vi "HCC Panel Get Cycle Count.vi"(0 "Main Washer Display In":T9={"Status Color"=0, "Station Label Display"="", "Cycle Count Display"=0, "Board ID Display"="", "Serial Number Display"="", "Current Display"=0.0, "RPM Display"=0, "Saving Display"=FALSE, "Appliance Details"={"FileVersionInfo"={"FileVersion"="", "ProductName"="", "InternalName"="", "CompanyName"="", "LegalCopyright"="", "FileDescription"=""}, "Dishwasher Info"={"Open Cup Weight (gm):"=0.0, "Auto Cup Weight (gm):"=0.0, "Detergent-Dish:"="", "Inlet Temperature-Dish:"="", "Cycle Mode-Dish:"="", "Unit Control-Dish:"="", "Manufacturer-Dish:"=""}, "Washer Info"={"Hot Water Temperature (Fahrenheit):"="", "Cold Water Temperature (Fahrenheit):"="", "Capacity (cu.ft):"=0.0, "Initial Cloth Weight:"=0.0, "Cloth Lot:"=0, "Model Family:"="", "Program Name:"="", "Cycle Selection:"="", "Wash Temperature:"="", "Rinse Temperature:"="", "Load Size:"=""}, "File Name Output Array"=[], "Calibration Output Array"=[], "Appliance Common"={"Engineer:"="", "Model Number:"="", "Serial Number:"="", "Comments:"="", "Station ID:"="", "Technician:"="", "TR Number:"="", "Lab ID:"="", "Voltage:"="", "Water Pressure (PSI):"="", "Test Date:"="", "Computer Name:"="", "IP Address:"="", "Ambient RH:"="", "Frequency:"="", "Build:"="", "Filename:"="", "Test Type:"="", "Load Run #:"=0, "Ambient Temperature (F):"="", "File Path:"=path ""}, "Water Heater"={"Heating Mode:"=""}, "Dryer"={"Heat Setting:"="", "Washer Water Temperature (60 ± 5°F):"=60, "Water Hardness (PPM):"=17, "Dryness Setting:"="", "Dryer Type:"="", "Exhaust:"="", "Drying Cycle:"="", "Load Type:"="", "Nominal Load Weight"="", "Dryer Initial IMC Data"={"Measured IMC"=7.0, "Actual RMC"=7.0, "RMC (Desired)"=100.0, "Bone Dry Wt(lbs)"=7.0, "Tolerance(%)"=5.0}, "Empty Dryer Cold Weigth"=60.0}}, "Current Run Start Time Display"=0.0, "UI Button"=FALSE, "Current Path Display"=path "", "Unit Type Display"=enum."", "Total Time On Display"=0.0, "Headers"={"Summary Header"=["Date", "Time", "Total Cycle Time (Seconds)", "Cycle Number", "Maximum RPM", "# of Error Codes", "Maximum Current"], "Current Header"=["Date", "Time", "Time (Seconds)", "Current (Amps)"], "Debug Log Header"=["Date", "Time", "Debug Logs"], "Data Header"=["Date", "Time", "Time (Seconds)", "IGBT Temperature", "Speed", "Load Size", "Temperature", "Water Pressure", "Detergent", "Fabric Softener", "Direction", "Detergent Valve", "Fabric Softener Valve", "Recirculating Pump", "Drain Valve", "Hot Water Valve", "Cold Water Valve", "Lid Status", "Lid Lock Status", "Machine Status", "Serial Number", "Cycle Count", "Station Label", "Board ID", "Error", "End of Cycle"]}} {"Appliance Details"."Dryer"."Dryer Initial IMC Data"."Tolerance(%)" format="%0#_6g"; "Appliance Details"."Dryer"."Dryer Initial IMC Data"."Bone Dry Wt(lbs)" format="%03_6g"; "Appliance Details"."Dryer"."Dryer Initial IMC Data"."RMC (Desired)" format="%0#_6g"; "Appliance Details"."Dryer"."Dryer Initial IMC Data"."Actual RMC" format="%03_6g"; "Appliance Details"."Dryer"."Dryer Initial IMC Data"."Measured IMC" format="%0#_6g"; "Current Display" format="%.2f"; "Cycle Count Display" format="%04d"}, 2 "GEA Information In":T1 {"Water Heater GEA2 Data"."Hyperterminal Data"."CRC" format="%x"; "Water Heater GEA2 Data"."Hyperterminal Data"."Length" format="%x"; "Water Heater GEA2 Data"."Hyperterminal Data"."Command" format="%x"; "Water Heater GEA2 Data"."Hyperterminal Data"."Destination" format="%x"; "Water Heater GEA2 Data"."Hyperterminal Data"."Source" format="%x"; "Destination Address" format="%x"; "Source Address" format="%x"; "Command" format="%.0x"; "Data to send" format="%x"; "ReceivedData" format="%x"}, 5 "error in (no error)":errorcluster) -> (14 "Main Washer Display Out":T9={"Status Color"=0, "Station Label Display"="", "Cycle Count Display"=0, "Board ID Display"="", "Serial Number Display"="", "Current Display"=0.0, "RPM Display"=0, "Saving Display"=FALSE, "Appliance Details"={"FileVersionInfo"={"FileVersion"="", "ProductName"="", "InternalName"="", "CompanyName"="", "LegalCopyright"="", "FileDescription"=""}, "Dishwasher Info"={"Open Cup Weight (gm):"=0.0, "Auto Cup Weight (gm):"=0.0, "Detergent-Dish:"="", "Inlet Temperature-Dish:"="", "Cycle Mode-Dish:"="", "Unit Control-Dish:"="", "Manufacturer-Dish:"=""}, "Washer Info"={"Hot Water Temperature (Fahrenheit):"="", "Cold Water Temperature (Fahrenheit):"="", "Capacity (cu.ft):"=0.0, "Initial Cloth Weight:"=0.0, "Cloth Lot:"=0, "Model Family:"="", "Program Name:"="", "Cycle Selection:"="", "Wash Temperature:"="", "Rinse Temperature:"="", "Load Size:"=""}, "File Name Output Array"=[], "Calibration Output Array"=[], "Appliance Common"={"Engineer:"="", "Model Number:"="", "Serial Number:"="", "Comments:"="", "Station ID:"="", "Technician:"="", "TR Number:"="", "Lab ID:"="", "Voltage:"="", "Water Pressure (PSI):"="", "Test Date:"="", "Computer Name:"="", "IP Address:"="", "Ambient RH:"="", "Frequency:"="", "Build:"="", "Filename:"="", "Test Type:"="", "Load Run #:"=0, "Ambient Temperature (F):"="", "File Path:"=path ""}, "Water Heater"={"Heating Mode:"=""}, "Dryer"={"Heat Setting:"="", "Washer Water Temperature (60 ± 5°F):"=60, "Water Hardness (PPM):"=17, "Dryness Setting:"="", "Dryer Type:"="", "Exhaust:"="", "Drying Cycle:"="", "Load Type:"="", "Nominal Load Weight"="", "Dryer Initial IMC Data"={"Measured IMC"=7.0, "Actual RMC"=7.0, "RMC (Desired)"=100.0, "Bone Dry Wt(lbs)"=7.0, "Tolerance(%)"=5.0}, "Empty Dryer Cold Weigth"=60.0}}, "Current Run Start Time Display"=0.0, "UI Button"=FALSE, "Current Path Display"=path "", "Unit Type Display"=enum."", "Total Time On Display"=0.0, "Headers"={"Summary Header"=["Date", "Time", "Total Cycle Time (Seconds)", "Cycle Number", "Maximum RPM", "# of Error Codes", "Maximum Current"], "Current Header"=["Date", "Time", "Time (Seconds)", "Current (Amps)"], "Debug Log Header"=["Date", "Time", "Debug Logs"], "Data Header"=["Date", "Time", "Time (Seconds)", "IGBT Temperature", "Speed", "Load Size", "Temperature", "Water Pressure", "Detergent", "Fabric Softener", "Direction", "Detergent Valve", "Fabric Softener Valve", "Recirculating Pump", "Drain Valve", "Hot Water Valve", "Cold Water Valve", "Lid Status", "Lid Lock Status", "Machine Status", "Serial Number", "Cycle Count", "Station Label", "Board ID", "Error", "End of Cycle"]}} {"Appliance Details"."Dryer"."Dryer Initial IMC Data"."Tolerance(%)" format="%0#_6g"; "Appliance Details"."Dryer"."Dryer Initial IMC Data"."Bone Dry Wt(lbs)" format="%03_6g"; "Appliance Details"."Dryer"."Dryer Initial IMC Data"."RMC (Desired)" format="%0#_6g"; "Appliance Details"."Dryer"."Dryer Initial IMC Data"."Actual RMC" format="%03_6g"; "Appliance Details"."Dryer"."Dryer Initial IMC Data"."Measured IMC" format="%0#_6g"; "Current Display" format="%.2f"; "Cycle Count Display" format="%04d"}, 16 "GEA Information Out":T1 {"Water Heater GEA2 Data"."Hyperterminal Data"."CRC" format="%x"; "Water Heater GEA2 Data"."Hyperterminal Data"."Length" format="%x"; "Water Heater GEA2 Data"."Hyperterminal Data"."Command" format="%x"; "Water Heater GEA2 Data"."Hyperterminal Data"."Destination" format="%x"; "Water Heater GEA2 Data"."Hyperterminal Data"."Source" format="%x"; "Destination Address" format="%x"; "Source Address" format="%x"; "Command" format="%.0x"; "Data to send" format="%x"; "ReceivedData" format="%x"}, 17 "GEA Ref Out":refnum<k24>, 18 "Event Registration Out":refnum<event-registration>, 19 "error out":errorcluster)   [LabVIEW 2014]
uses:
  Utility/Save File/Public/Type Definitions/Save File Washer.ctl
  Utility/Save File/File Setup (Public)/Type Definition/Save File DISH Dishwasher Details.ctl
  <vilib>/Platform/fileVersionInfo.llb/FileVersionInformation.ctl
  Utility/Custom Pallet Controls/Custom Pallet String.ctl
  Utility/Save File/Public/Type Definitions/Save File Unit Type.ctl
  Utility/Save File/Public/Type Definitions/Save File Headers.ctl
  Type Definitions/ViperHawk/ViperHawk Data.ctl
  Type Definitions/ViperHawk/ViperHawk Diagnostic Data.ctl
  Utility/Save File/Public/Type Definitions/Save File Software Version.ctl
  Type Definitions/ViperHawk/ViperHawk Search Control.ctl
  C:/Technology Lab/NI-2010/Trunk/Utility/LabVIEW GEA2 Toolkit v1.0.0.0/Appliance.NET/GeaCommunication.dll
  Utility/LabVIEW GEA2 Toolkit v1.0.0.0/Appliance.NET/GeaCommunication.dll
  Utility/LabVIEW GEA2 Toolkit v1.0.0.0/type defs/Data Out.ctl
  Utility/GEA2 Commands/HEWH/Type Definitions/GEA2 Commands WaterHeater GEA2 Data.ctl
  Utility/GEA2 Commands/HEWH/Type Definitions/GEA2 Commands Button Status.ctl
  Utility/GEA2 Commands/HEWH/Type Definitions/GEA2 Commands Status Query.ctl
  Utility/GEA2 Commands/HEWH/Type Definitions/GEA2 Commands Service Error Codes.ctl
  Utility/LabVIEW GEA2 Toolkit v1.0.0.0/type defs/ERD Read Data In.ctl
  Utility/LabVIEW GEA2 Toolkit v1.0.0.0/type defs/Data Type.ctl
  Utility/LabVIEW GEA2 Toolkit v1.0.0.0/type defs/Source_Destination.ctl
  Utility/LabVIEW GEA2 Toolkit v1.0.0.0/type defs/Data In.ctl
  Utility/LabVIEW GEA2 Toolkit v1.0.0.0/library/GEA2_Toolkit.lvlib
  Utility/Save File/Save File.lvlib
  Utility/Save File/File Setup.lvlib
panel:
  out "Total Cycle Count":u16
  in  "Complete":bool
  in  "String":string="Finding Machine Cycle Count"
  in  "Tab Control":enum32{"Page 1"}(tab)
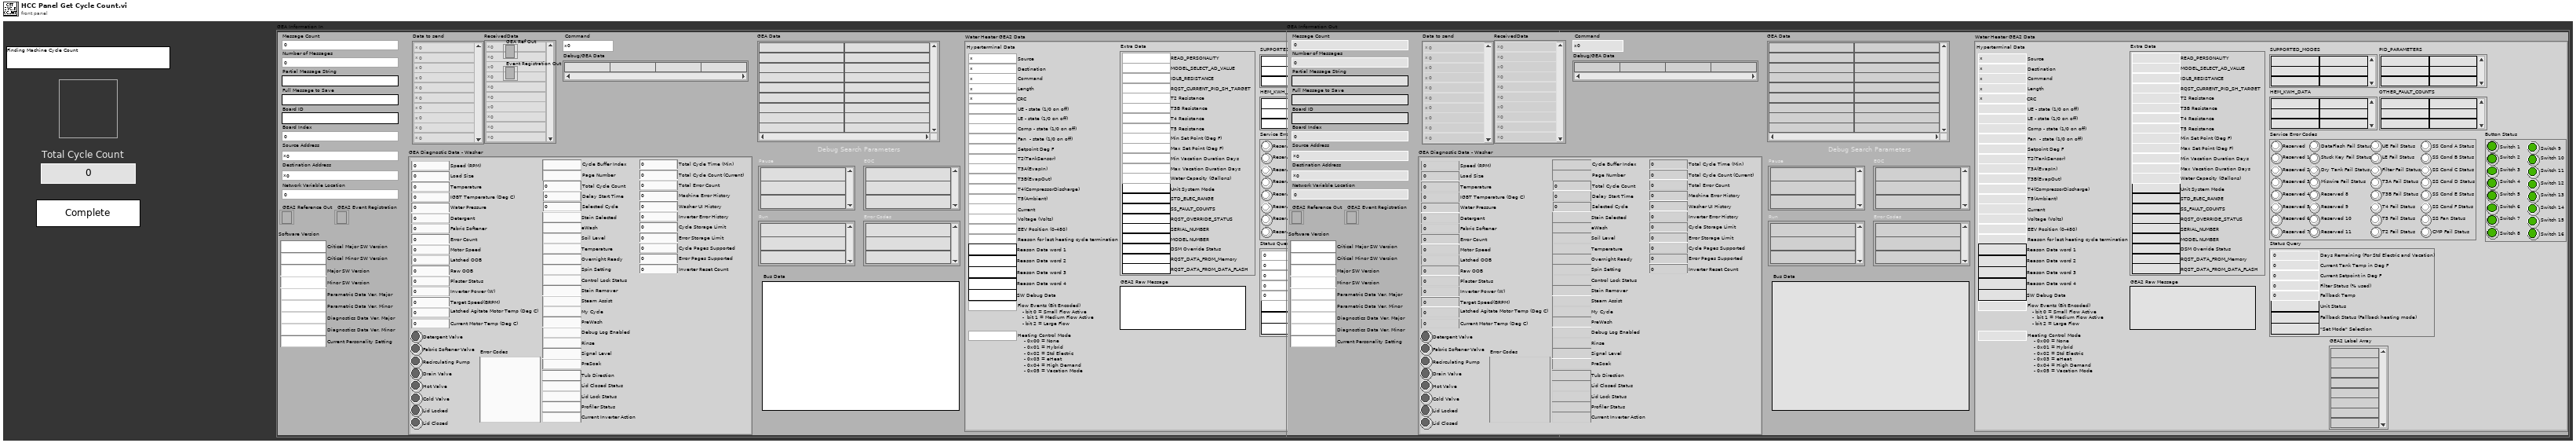
[diagram p1: front panel]
types:
  T1 = typedef "ViperHawk Data.ctl" = cluster{"GEA Diagnostic Data - Washer":T2, "Software Version":T3, "Debug Search Parameters":T4, "Message Count":i32, "Number of Messages":i32, "Partial Message String":string, "Full Message to Save":string, "Board ID":string, "Board Index":i32, "Source Address":u8, "Destination Address":u8, "Data to send":u8[], "ReceivedData":u8[], "Debug/GEA Data":string[], "Command":u8, "GEA2 Reference Out":refnum<k24>, "GEA2 Event Registration":refnum<event-registration>, "Bus Data":string, "GEA Data":string[][], "Network Variable Location":i32, "Water Heater GEA2 Data":T5}
  T2 = typedef "ViperHawk Diagnostic Data.ctl" = cluster{"Speed (RPM)":u32, "Load Size":u32, "Temperature":u32, "Water Pressure":u32, "Detergent":u32, "Fabric Softener":u32, "Tub Direction":string, "Detergent Valve":bool, "Fabric Softener Valve":bool, "Recirculating Pump":bool, "Drain Valve":bool, "Hot Valve":bool, "Cold Valve":bool, "Lid Closed Status":string, "Lid Lock Status":string, "Error Count":u32, "IGBT Temperature (Deg C)":u32, "Motor Speed":u32, "Latched OOB":u32, "Raw OOB":u32, "Plaster Status":u32, "Inverter Power (W)":u32, "Target Speed(BRPM)":u32, "Latched Agitate Motor Temp (Deg C)":u32, "Current Motor Temp (Deg C)":u32, "Profiler Status":string, "Current Inverter Action":string, "Error Codes":string, "Lid Locked":bool, "Lid Closed":bool, "9E Diagnostic Data":cluster{"Total Cycle Time (Min)":u32, "Total Cycle Count (Current)":u16, "Total Error Count":u16, "Machine Error History":u32, "Washer UI History":u32, "Inverter Error History":u32, "Cycle Storage Limit":u8, "Error Storage Limit":u8, "Cycle Pages Supported":u8, "Error Pages Supported":u8, "Inverter Reset Count":u16}, "9F Diagnostic Data":cluster{"Cycle Buffer Index":string, "Page Number":string, "Total Cycle Count":u32, "Delay Start Time":u32, "Stain Selected":string, "Selected Cycle":u32, "eWash":string, "Soil Level":string, "Temperature":string, "Overnight Ready":string, "Spin Setting":string, "Control Lock Status":string, "Stain Remover":string, "Steam Assist":string, "My Cycle":string, "PreWash":string, "Debug Log Enabled":string, "Rinse":string, "Signal Level":string, "PreSoak":string}}
  T3 = typedef "Save File.lvlib/Save File Software Version.ctl" = cluster{"Critical Major SW Version":string, "Critical Minor SW Version":string, "Major SW Version":string, "Minor SW Version":string, "Parametric Data Ver. Major":string, "Parametric Data Ver. Minor":string, "Diagnostics Data Ver. Major":string, "Diagnostics Data Ver. Minor":string, "Current Personality Setting":string}
  T4 = typedef "ViperHawk Search Control.ctl" = cluster{"Pause":string[], "Run":string[], "EOC":string[], "Error Codes":string[]}
  T5 = typedef "GEA2 Commands WaterHeater GEA2 Data.ctl" = cluster{"GEA2 Label Array":string[], "PID_PARAMETERS":string[][], "SUPPORTED_MODES":string[][], "Button Status":T6, "Status Query":T7, "Service Error Codes":T8, "HEM_KWH_DATA":string[][], "OTHER_FAULT_COUNTS":string[][], "GEA2 Raw Message":string, "Hyperterminal Data":cluster{"Source":u8, "Destination":u8, "Command":u8, "Length":u8, "CRC":u16, "UE - state (1/0 on off)":u8, "LE - state (1/0 on off)":u8, "Comp - state (1/0 on off)":u8, "Fan  - state (1/0 on off)":u8, "Setpoint Deg F":i32, "T2(TankSensor)":dbl, "T3A(EvapIn)":dbl, "T3B(EvapOut)":dbl, "T4(CompressorDischarge)":dbl, "T5(Ambient)":dbl, "Current":dbl, "Voltage (Volts)":u16, "EEV Position (0-480)":u16, "Reason for last heating cycle termination":u16, "Reason Data word 1":string, "Reason Data word 2":string, "Reason Data word 3":string, "Reason Data word 4":string, "SW Debug Data":string, "Flow Events (Bit Encoded)":u16, "Heating Control Mode":u16}, "Extra Data":cluster{"Water Capacity (Gallons)":u32, "Max Vacation Duration Days":u32, "Min Vacation Duration Days":u32, "Max Set Point (Deg F)":u32, "Min Set Point (Deg F)":u32, "T5 Resistance":u32, "T4 Resistance":u32, "T3B Resistance":u32, "T2 Resistance":u32, "STD_ELEC_RANGE":string, "SS_FAULT_COUNTS":string, "SERIAL_NUMBER":string, "READ_PERSONALITY":u8, "RQST_OVERRIDE_STATUS":string, "MODEL_SELECT_AD_VALUE":u32, "MODEL NUMBER":string, "IDLB_RESISTANCE":u32, "DSM Override Status":string, "RQST_DATA_FROM_Memory":string, "RQST_DATA_FROM_DATA_FLASH":string, "RQST_CURRENT_PID_SH_TARGET":u16, "Unit System Mode":string}}
  T6 = typedef "GEA2 Commands Button Status.ctl" = cluster{"Switch 1":bool, "Switch 2":bool, "Switch 3":bool, "Switch 4":bool, "Switch 5":bool, "Switch 6":bool, "Switch 7":bool, "Switch 8":bool, "Switch 9":bool, "Switch 10":bool, "Switch 11":bool, "Switch 12":bool, "Switch 13":bool, "Switch 14":bool, "Switch 15":bool, "Switch 16":bool}
  T7 = typedef "GEA2 Commands Status Query.ctl" = cluster{"Days Remaining (For Std Electric and Vacation)":u8, "Unit Status":string, "Current Tank Temp in Deg F":u8, "Current Setpoint in Deg F":u8, "Filter Status (% used)":u8, "Fallback Status (Fallback heating mode)":string, "Fallback Temp":u8, "\"Set Mode\" Selection":string}
  T8 = typedef "GEA2 Commands Service Error Codes.ctl" = cluster{"Reserved":bool, "Reserved 1":bool, "Reserved 2":bool, "Reserved 3":bool, "Reserved 4":bool, "Reserved 5":bool, "Reserved 6":bool, "Reserved 7":bool, "DataFlash Fail Status":bool, "Stuck Key Fail Status":bool, "Dry Tank Fail Status":bool, "Miswire Fail Status":bool, "Reserved 8":bool, "Reserved 9":bool, "Reserved 10":bool, "Reserved 11":bool, "UE Fail Status":bool, "LE Fail Status":bool, "Filter Fail Status":bool, "T3A Fail Status":bool, "T3B Fail Status":bool, "T4 Fail Status":bool, "T5 Fail Status":bool, "T2 Fail Status":bool, "SS Cond A Status":bool, "SS Cond B Status":bool, "SS Cond C Status":bool, "SS Cond D Status":bool, "SS Cond E Status":bool, "SS Cond F Status":bool, "SS Fan Status":bool, "CMP Fail Status":bool}
  T9 = typedef "Save File.lvlib/Save File Washer.ctl" = cluster{"Status Color":u32, "Station Label Display":string, "Cycle Count Display":i32, "Board ID Display":string, "Serial Number Display":string, "Current Display":dbl, "RPM Display":u32, "Saving Display":bool, "Appliance Details":T10, "Current Run Start Time Display":dbl, "UI Button":bool, "Current Path Display":path, "Unit Type Display":T13, "Total Time On Display":dbl, "Headers":T14}
  T10 = typedef "File Setup.lvlib/Save File DISH Dishwasher Details.ctl" = cluster{"FileVersionInfo":T11, "Dishwasher Info":cluster{"Open Cup Weight (gm):":dbl, "Auto Cup Weight (gm):":dbl, "Detergent-Dish:":string, "Inlet Temperature-Dish:":string, "Cycle Mode-Dish:":string, "Unit Control-Dish:":string, "Manufacturer-Dish:":string}, "Washer Info":cluster{"Hot Water Temperature (Fahrenheit):":string, "Cold Water Temperature (Fahrenheit):":string, "Capacity (cu.ft):":dbl, "Initial Cloth Weight:":dbl, "Cloth Lot:":i32, "Model Family:":string, "Program Name:":string, "Cycle Selection:":string, "Wash Temperature:":string, "Rinse Temperature:":string, "Load Size:":string}, "File Name Output Array":string[][], "Calibration Output Array":string[][], "Appliance Common":cluster{"Engineer:":string, "Model Number:":string, "Serial Number:":string, "Comments:":string, "Station ID:":string, "Technician:":string, "TR Number:":string, "Lab ID:":string, "Voltage:":string, "Water Pressure (PSI):":string, "Test Date:":string, "Computer Name:":string, "IP Address:":string, "Ambient RH:":string, "Frequency:":string, "Build:":string, "Filename:":string, "Test Type:":string, "Load Run #:":i32, "Ambient Temperature (F):":string, "File Path:":path}, "Water Heater":cluster{"Heating Mode:":string}, "Dryer":cluster{"Heat Setting:":T12, "Washer Water Temperature (60 ± 5°F):":u16, "Water Hardness (PPM):":u16, "Dryness Setting:":T12, "Dryer Type:":string, "Exhaust:":string, "Drying Cycle:":string, "Load Type:":string, "Nominal Load Weight":string, "Dryer Initial IMC Data":cluster{"Measured IMC":dbl, "Actual RMC":dbl, "RMC (Desired)":dbl, "Bone Dry Wt(lbs)":dbl, "Tolerance(%)":dbl}, "Empty Dryer Cold Weigth":dbl}}
  T11 = typedef "FileVersionInformation.ctl" = cluster{"FileVersion":string, "ProductName":string, "InternalName":string, "CompanyName":string, "LegalCopyright":string, "FileDescription":string}
  T12 = typedef "Custom Pallet String.ctl" = string
  T13 = typedef "Save File.lvlib/Save File Unit Type.ctl" = enum32{"", "Viper", "Hawk", "2015", "HEWH", "Other"}
  T14 = typedef "Save File Headers.ctl" = cluster{"Summary Header":string[], "Current Header":string[], "Debug Log Header":string[], "Data Header":string[]}
  T15 = typedef "GEA2_Toolkit.lvlib/Data In.ctl" = cluster{"Source":u8, "Destination":u8, "Command":u8, "Message":string}
  T16 = typedef "GEA2_Toolkit.lvlib/Source_Destination.ctl" = cluster{"Source":u8, "Destination":u8}
  T17 = typedef "GEA2_Toolkit.lvlib/ERD Read Data In.ctl" = cluster{"ERD Number":u16, "Data Type":T18}
  T18 = typedef "GEA2_Toolkit.lvlib/Data Type.ctl" = enum16{"string", "boolean", "uint8_t", "uint16_t", "uint32_t", "uint64_t"}
  T19 = typedef "GEA2_Toolkit.lvlib/ERD Read Data Out.ctl" = cluster{"ERD Number":u16, "Data":string}
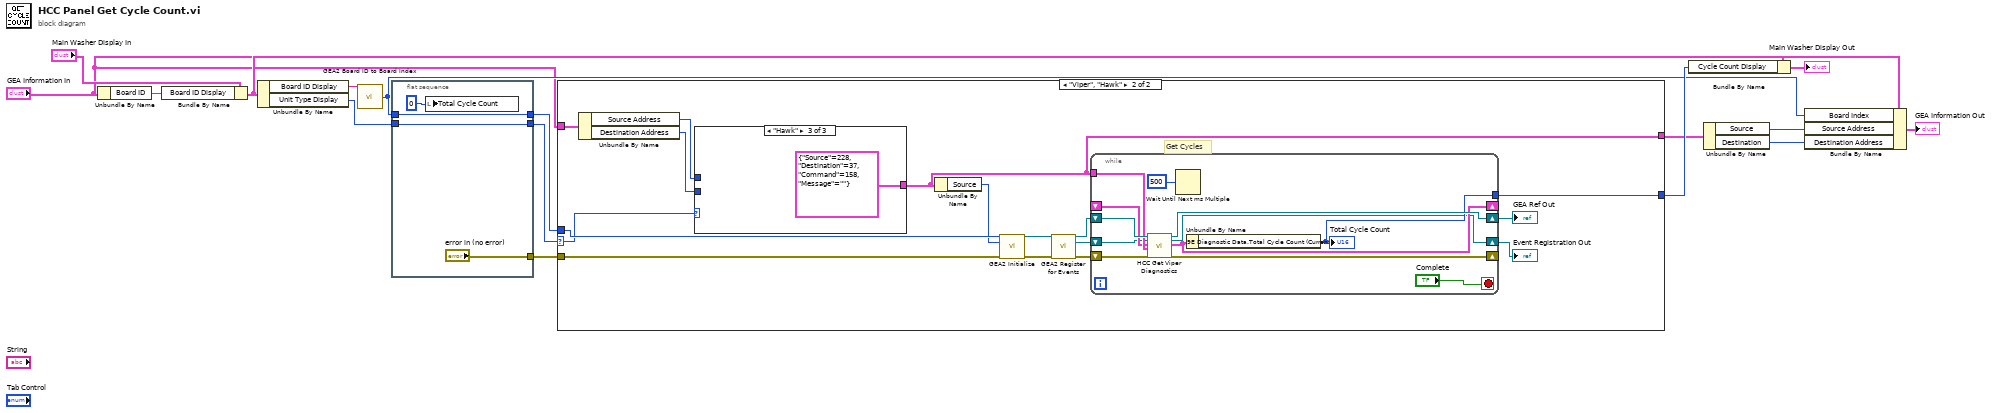
[diagram p0: block diagram]
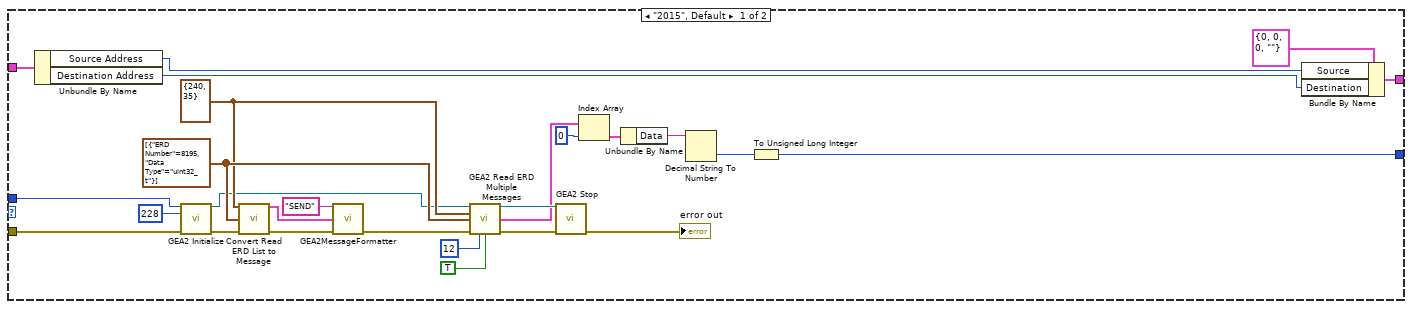
[diagram p2: hidden frame]
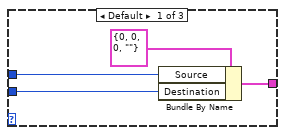
[diagram p3: hidden frame]
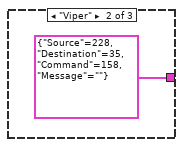
[diagram p4: hidden frame]
diagram:
  n1 = Unbundle By Name("GEA Information In") -> ("Board ID"=w8:string)
  n2 = Bundle By Name(cluster="Main Washer Display In", "Board ID Display"=w8) -> (w7:T9)
  n3 = Unbundle By Name(w7) -> ("Board ID Display"=w13:string, "Unit Type Display"=w12:T13)
  n4 = call "GEA2 Board ID to Board Index.vi"("Board ID"=w13) -> ("Board Index"=w6:i32)  [unwired: 10 in, 4 out]
  n5 = flat-sequence {
    tunnel: [w17] -> w16
    tunnel: ["error in (no error)"] -> w15
    tunnel: [w18] -> w14
    tunnel: w6 -> [w18]
    tunnel: w12 -> [w17]
    frame #0 {
      n6 = local write "Total Cycle Count"(u16 0 ("Total Cycle Count")) -> ()
    }
  }
  n7 = case shown="\"Viper\", \"Hawk\"" w16 {
    selector: w16 -> [_ w61]
    tunnel: w15 -> [w35 w63]
    tunnel: w14 -> [w34 w62]
    tunnel: [w26 w59] -> w11
    tunnel: "GEA Information In" -> [w25 w51]
    tunnel: [w21 w48] -> w3
    frame "2015", Default {
      w46 = T16 {"Source"=240, "Destination"=35} ("GEA Inputs")
      w47 = T17[] [{"ERD Number"=8195, "Data Type"=enum."uint32_t"}]
      n8 = Unbundle By Name(w25) -> ("Source Address"=w23:u8, "Destination Address"=w22:u8)
      n9 = call "GEA2 Initialize.vi"("Board Index"=w34, "Source Address"=u8 228, "error in"=w35) -> ("GEA2 Reference Out"=w38:refnum<k24>, "error out"=w43:errorcluster)  [unwired: 10 in, 1 out]
      n10 = call "Convert Read ERD List to Message.vi"("GEA Inputs"=w46, "Read ERD List"=w47, "Error In"=w43) -> ("GEA Message"=w37:T15, "Error Out"=w41:errorcluster)  [unwired: 11 in]
      n11 = call "GEA2MessageFormatter.vi"("Prefix(Send/Recv)"="SEND", "GEA2 Data In"=w37, "Error In"=w41) -> ("Error Out"=w42:errorcluster)  [unwired: 11 in, 1 out]
      n12 = call "GEA2 Read ERD Multiple Messages.vi"("GEA2 Reference In"=w38, "GEA Inputs"=w46, "Read ERD List"=w47, "Error In"=w42, "#ERDs per message"=12, "Verify ERD Response?"=TRUE) -> ("GEA2 Reference Out"=w44:refnum<k24>, "ERD Data Out"=w31:T19[], "Error Out"=w32:errorcluster)  [unwired: 5 in, 2 out]
      n13 = call "GEA2 Stop.vi"("GEA2 Reference Out"=w44, "Error In"=w32) -> ("Error Out"=→"error out":errorcluster)  [unwired: 13 in]
      n14 = Index Array(array=w31, index=0) -> (element=w29:T19)
      n15 = Unbundle By Name(w29) -> ("Data"=w27:string)
      n16 = Decimal String To Number(string=w27) -> (number=w28:i32)  [unwired: 2 in, 1 out]
      n17 = To Unsigned Long Integer(number=w28) -> (unsigned 32bit integer=w26:u32)
      n18 = Bundle By Name(cluster=T15 {"Source"=0, "Destination"=0, "Command"=0, "Message"=""} ("Input Data"), "Source"=w23, "Destination"=w22) -> (w21:T15)
    }
    frame "Viper", "Hawk" {
      # "Get Cycles"
      n19 = Unbundle By Name(w51) -> ("Source Address"=w50:u8, "Destination Address"=w49:u8)
      n20 = case shown="\"Hawk\"" w61 {
        tunnel: [w66 T15 {"Source"=228, "Destination"=35, "Command"=158, "Message"=""} ("Input Data") T15 {"Source"=228, "Destination"=37, "Command"=158, "Message"=""} ("Input Data")] -> w48
        tunnel: w50 -> [w65 _ _]
        tunnel: w49 -> [w64 _ _]
        frame Default {
          n21 = Bundle By Name(cluster=T15 {"Source"=0, "Destination"=0, "Command"=0, "Message"=""} ("Input Data"), "Source"=w65, "Destination"=w64) -> (w66:T15)
        }
        frame "Viper" {
        }
        frame "Hawk" {
        }
      }
      n22 = Unbundle By Name(w48) -> ("Source"=w60:u8)
      n23 = call "GEA2 Initialize.vi"("Board Index"=w62, "Source Address"=w60, "error in"=w63) -> ("GEA2 Reference Out"=w56:refnum<k24>, "error out"=w53:errorcluster)  [unwired: 10 in, 1 out]
      n24 = call "GEA2 Register for Events.vi"("GEA2 Reference In"=w56, "Error In"=w53) -> ("GEA2 Reference Out"=w55:refnum<k24>, "GEA2 Event Registration"=w54:refnum<event-registration>, "Error Out"=w52:errorcluster)  [unwired: 11 in]
      n25 = while {
        tunnel: w48 -> [w76]
        shift-right: [w77] -> w57
        shift-left: w55 -> [w78]
        shift-right: [w79] -> _
        shift-left: w52 -> [w80]
        shift-right: [w74] -> _
        shift-left: _ -> [w75]
        tunnel: [w73] -> w59
        shift-right: [w70] -> w58
        shift-left: w54 -> [w71]
        stop <- "Complete" stop-if-true
        n26 = call "HCC Get Viper Diagnostics.vi"("GEA Ref In"=w78, "GEA2 Event Registration"=w71, "Diagnostic"=w75, "Input Data"=w76, "error in (no error)"=w80) -> ("GEA Ref Out"=w77:refnum<k24>, "Event Registration Out"=w70:refnum<event-registration>, "Diagnostic Data Output"=w74:T2, "error out"=w79:errorcluster)  [unwired: 10 in, 1 out]
        n27 = Wait Until Next ms Multiple(millisecond multiple=u32 500) -> ()  [unwired: 1 out]
        n28 = Unbundle By Name(w74) -> ("9E Diagnostic Data.Total Cycle Count (Current)"=w73:u16)
        "Total Cycle Count" <- w73
      }
      "Event Registration Out" <- w58
      "GEA Ref Out" <- w57
    }
  }
  n29 = Bundle By Name(cluster=w7, "Cycle Count Display"=w11) -> (→"Main Washer Display Out":T9)
  n30 = Unbundle By Name(w3) -> ("Source"=w2:u8, "Destination"=w1:u8)
  n31 = Bundle By Name(cluster="GEA Information In", "Board Index"=w6, "Source Address"=w2, "Destination Address"=w1) -> (→"GEA Information Out":T1)
